vi "Show or Hide Module.vi"(10 "long width":u32=272, 11 "Connections Reference":refnum<vi>) -> ()   [LabVIEW 2017]
panel:
  in  "show Module":bool
  in  "Connections":T1(array[cluster])
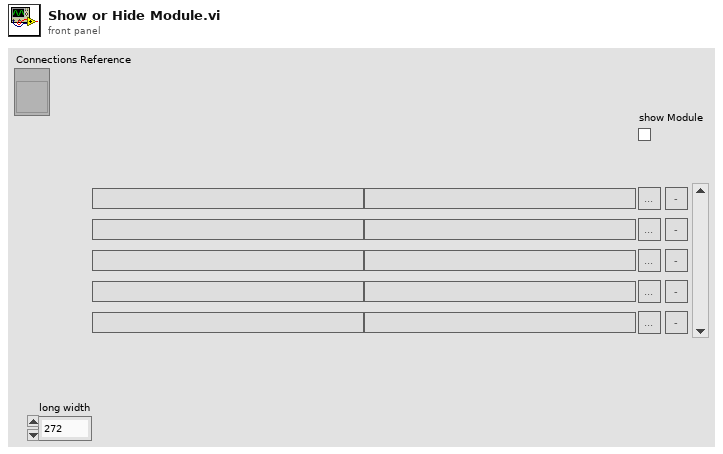
[diagram p1: front panel]
types:
  T1 = cluster{"Module":string, "Source":string, "Destination":string, "Edit":bool, "Remove":bool}[]
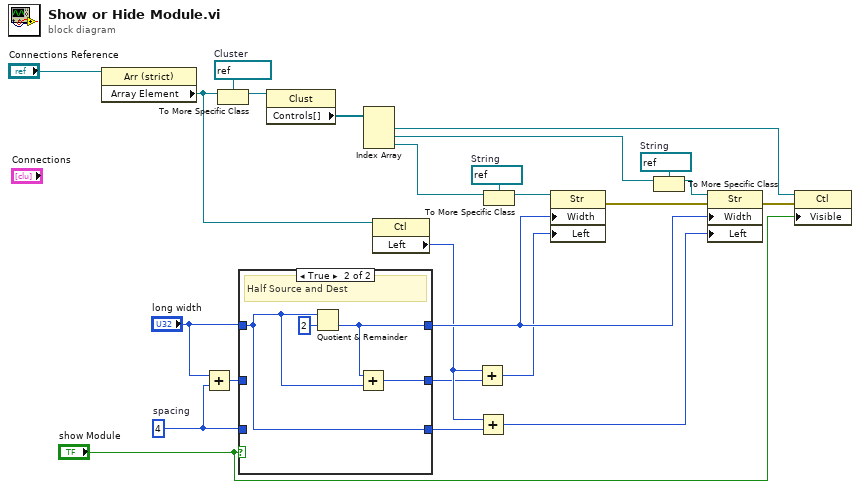
[diagram p0: block diagram]
diagram:
  w4 = u32 4  # spacing
  w16 = refnum<vi> refnum  # String
  w21 = refnum<vi> refnum  # String
  w24 = refnum<vi> refnum  # Cluster
  n1 = property class="Arr (strict)"(reference="Connections Reference") -> ("Array Element"=w12:refnum<vi>)  [unwired: 1 in, 2 out]
  n2 = Add(x="long width", y=w4) -> (x+y=w2:u32)
  n3 = To More Specific Class(target class=w24, reference=w12) -> (specific class reference=w13:refnum<vi>)  [unwired: 1 in, 1 out]
  n4 = case shown="True" "show Module" {
    tunnel: "long width" -> [w27 w29]
    tunnel: [w27 w30] -> w10
    tunnel: w4 -> [w26 _]
    tunnel: [w26 w29] -> w9
    tunnel: [w25 w28] -> w6
    tunnel: w2 -> [w25 _]
    frame False {
      # "Full Source and Dest"
    }
    frame True {
      # "Half Source and Dest"
      n5 = Quotient & Remainder(x=w29, y=u32 2) -> (floor(x/y)=w30:u32)  [unwired: 1 out]
      n6 = Add(x=w30, y=w29) -> (x+y=w28:u32)
    }
  }
  n7 = property class="Clust"(reference=w13) -> ("Controls[]"=w23:refnum<vi>[])  [unwired: 1 in, 2 out]
  n8 = Index Array(array=w23) -> (element #1=w22:refnum<vi>, element #2=w20:refnum<vi>, element #3=w15:refnum<vi>)  [unwired: 3 in]
  n9 = property class="Ctl"(reference=w12) -> ("Left"=w7:i32)  [unwired: 1 in, 2 out]
  n10 = Add(x=w7, y=w6) -> (x+y=w5:u32)
  n11 = Add(x=w7, y=w9) -> (x+y=w8:u32)
  n12 = To More Specific Class(target class=w16, reference=w15) -> (specific class reference=w17:refnum<vi>)  [unwired: 1 in, 1 out]
  n13 = property class="Str"(reference=w17, "Width"=w10, "Left"=w5) -> (error out=w14:errorcluster)  [unwired: 1 in, 1 out]
  n14 = To More Specific Class(target class=w21, reference=w20) -> (specific class reference=w19:refnum<vi>)  [unwired: 1 in, 1 out]
  n15 = property class="Str"(reference=w19, error in=w14, "Width"=w10, "Left"=w8) -> (error out=w18:errorcluster)  [unwired: 1 out]
  n16 = property class="Ctl"(reference=w22, error in=w18, "Visible"="show Module") -> ()  [unwired: 2 out]
